vi "PDC_TriggerIn.vi"(8 "error in (no error)":errorcluster, 11 "DeviceNo":u32) -> (0 "error out":errorcluster, 3 "ReturnValue":u32, 4 "ErrorCode":u32)   [LabVIEW 2015]
doc: "This VI starts recording in the specified device."
uses:
  PDCLIB.dll
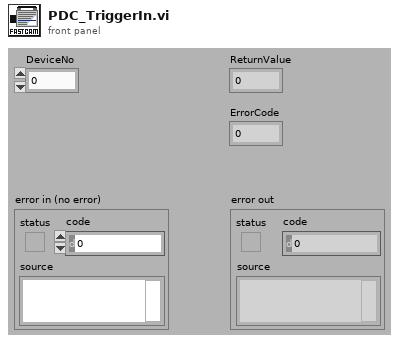
[diagram p1: front panel]
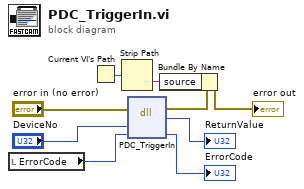
[diagram p0: block diagram]
diagram:
  n1 = local read "ErrorCode"() -> (w6:u32)
  n2 = Current VI's Path() -> (path=w3:path)
  n3 = Strip Path(path=w3) -> (name=w4:string)  [unwired: 1 out]
  n4 = dll-call lib="PDCLIB.dll" fn="PDC_TriggerIn"(error in="error in (no error)", "nDeviceNo"="DeviceNo", "pErrorCode"=w6) -> (error out=w2:errorcluster, "return type"=→"ReturnValue":u32, "pErrorCode"=→"ErrorCode":u32)  [unwired: 3 in, 1 out]
  n5 = Bundle By Name(cluster=w2, "source"=w4) -> (→"error out":errorcluster)
